vi "Detemine Multiplier Value.vi"(4 "Multiplier":T1) -> (1 "Numeric":dbl)   [LabVIEW 2018]
uses:
  Multiplier--control.ctl
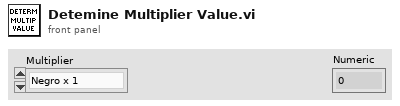
[diagram p1: front panel]
types:
  T1 = typedef "Multiplier--control.ctl" = enum16{"Negro x 1", "Marron x 10", "Rojo x 100", "Naranja x 1K", "Amarillo x 10K", "Verde x 100K", " Azul x 1M", "Violeta x 10M ", "Oro x 0.1", "Plata x 0.01"}
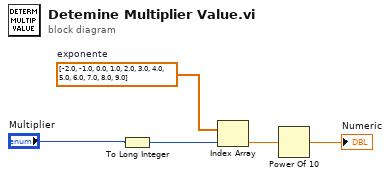
[diagram p0: block diagram]
diagram:
  w3 = dbl[] [-2.0, -1.0, 0.0, 1.0, 2.0, 3.0, 4.0, 5.0, 6.0, 7.0, 8.0, 9.0]  # exponente
  n1 = To Long Integer(number="Multiplier") -> (32bit integer=w4:i32)
  n2 = Index Array(array=w3, index=w4) -> (element=w2:dbl)
  n3 = Power Of 10(x=w2) -> (10^x=→"Numeric":dbl)
